vi "Create Mock.vi"(7 "VI Name":string, 8 "error in (no error)":errorcluster, 9 "Control value":variant[](array[variant]), 10 "Control Label":string[](array[string])) -> (0 "error out":errorcluster, 3 "Mock VI Call Out":refnum<class "Mock VI Call.lvclass">)   [LabVIEW 2020, in "Mock VI Call.lvclass"]
uses:
  Mock VI Call.lvclass
  Mock VI Call.lvclass/Mock VI Call.ctl
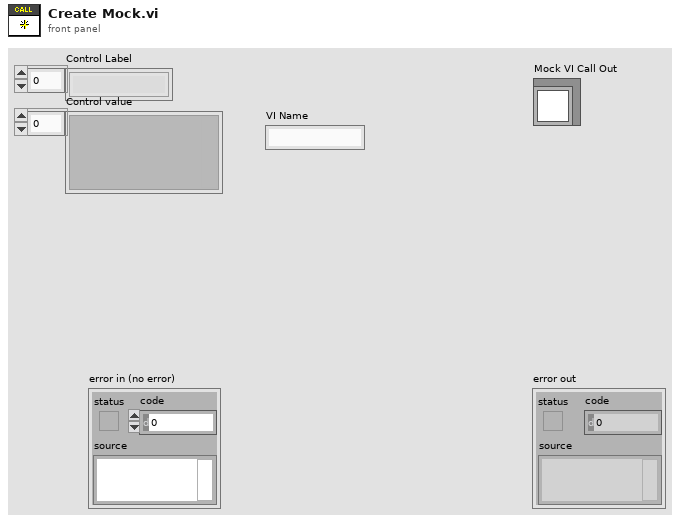
[diagram p1: front panel]
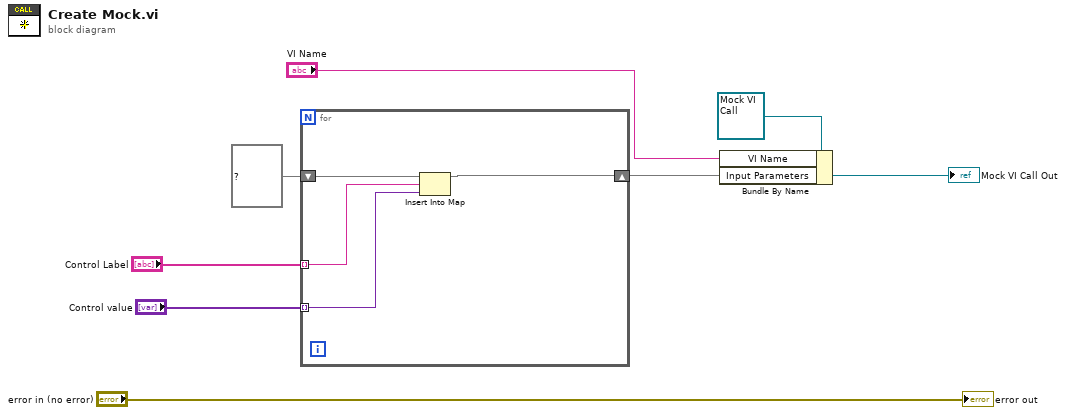
[diagram p0: block diagram]
diagram:
  n1 = for {
    tunnel: "Control Label" -> [w10] mode=indexing
    tunnel: "Control value" -> [w9] mode=indexing
    shift-right: [w11] -> w4
    shift-left: map{string, variant} {} ("Input Parameters") -> [w12]
    n2 = Insert Into Map(map in=w12, key=w10, value=w9) -> (map out=w11:map{string, variant})  [unwired: 2 out]
  }
  n3 = Bundle By Name(cluster=refnum<class "Mock VI Call.lvclass"> refnum ("Mock VI Call in"), "VI Name"="VI Name", "Input Parameters"=w4) -> (→"Mock VI Call Out":refnum<class "Mock VI Call.lvclass">)
  "error out" <- "error in (no error)"
